vi "Multicast SubVI.vi"() -> (2 "nDevices":i32 caption="Найдено устройств", 3 "str":string[](array[string]))   [LabVIEW 2017, in "LV_Unicorn.lvlib"]
uses:
  LV_Unicorn.lvlib
  <vilib>/Utility/error.llb/DialogType.ctl
  Control/AnswerUDP.ctl
  GlobalMulticast.vi
  <vilib>/Utility/tcp.llb/UDP Multicast Read-Write Open.vi
panel:
  out "Array":string[][](array[string])
  out "modbustype, version":u32=4294967295 format="%08x"
  out "net address":u32
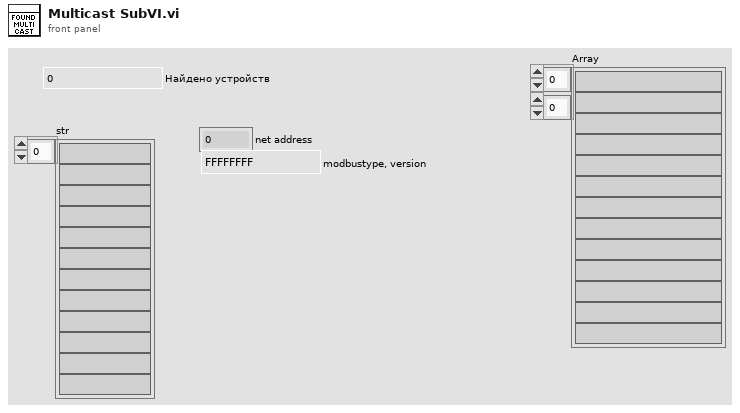
[diagram p1: front panel]
types:
  T1 = typedef "LV_Unicorn.lvlib/AnswerUDP.ctl" = cluster{"IP":string, "Port":u16, "DataVersion":u16, "ModbusAddress":i32, "type_version":string, "Description":string, "Serial":string, "ServerPort":u16}
  T2 = typedef "DialogType.ctl" = u16
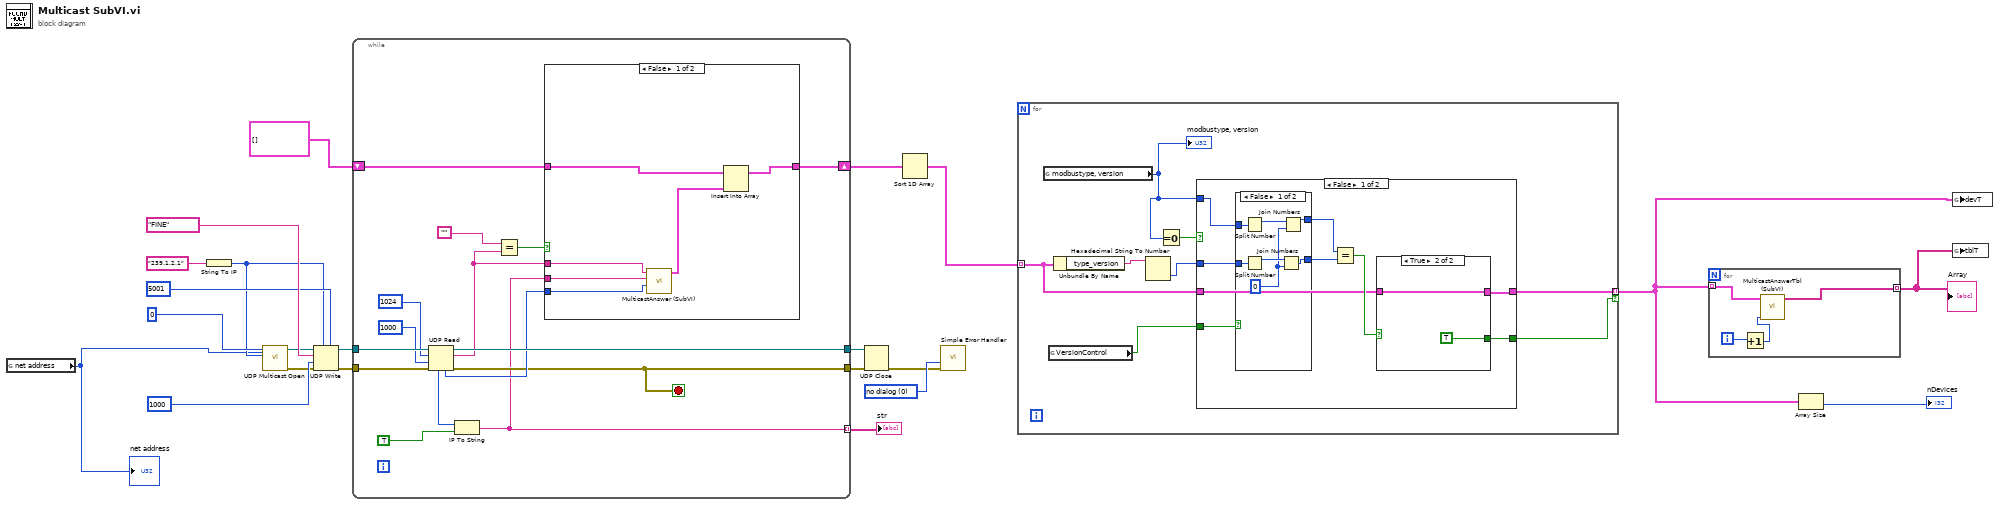
[diagram p0: block diagram]
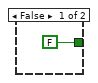
[diagram p3: hidden frame]
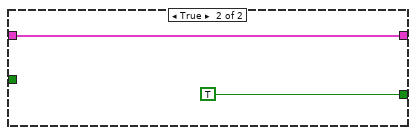
[diagram p4: hidden frame]
diagram:
  w17 = T2 0 items=["no dialog", "OK message", "continue or stop message", "OK message + warnings", "continue/stop + warnings"] ("type of dialog (OK msg:1)")
  n1 = global read "GlobalMulticast.vi" "net address"() -> (w1:u32)
  "net address" <- w1
  n2 = String To IP(1:"239.1.2.1" ("address")) -> (0:w12:u32)
  n3 = call-poly <vilib>:"UDP Multicast Open.vi"("net address"=w1, "multicast addr"=w12, "port"=u16 0) -> ("error out"=w13:errorcluster, "connection ID"=w14:refnum<k16>)  [unwired: 6 in, 1 out]
  n4 = UDP Write(address=w12, port or service name=u16 5001 ("port"), connection ID=w14, data in="FINE", 8:w13, 9:1000 ("timeout ms (25000)")) -> (error out=w9:errorcluster, 3:w11:refnum<k16>)
  n5 = while {
    tunnel: w11 -> [w37]
    tunnel: [w36] -> w10
    tunnel: w9 -> [w35]
    tunnel: [w28] -> w8
    tunnel: [w25] -> w22 mode=indexing
    shift-right: [w24] -> w7
    shift-left: T1[] [] -> [w23]
    stop <- w28 stop-if-true
    n6 = UDP Read(connection ID=w37, max size (548)=1024, timeout ms (25000)=1000, 8:w35) -> (data out=w31:string, error out=w28:errorcluster, 3:w36:refnum<k16>, 4:w30:u16, 6:w27:u32)
    n7 = IP To String(1:TRUE ("dot notation? (F)"), 2:w27) -> (0:w25:string)
    n8 = Equal?(x="", y=w31) -> (x = y?=w33:bool)
    n9 = case shown="False" w33 {
      tunnel: w31 -> [w43 _]
      tunnel: w25 -> [w42 _]
      tunnel: w30 -> [w41 _]
      tunnel: [w40 w44] -> w24
      tunnel: w23 -> [w39 w44]
      frame False {
        n10 = call "MulticastAnswer (SubVI).vi"("port"=w41, "name"=w42, "data in"=w43) -> ("SUdpAnswer"=w38:T1)  [unwired: 7 in, 1 out]
        n11 = Insert Into Array(array=w39, new element=w38) -> (w40:T1[])  [unwired: 1 in]
      }
      frame True {
      }
    }
  }
  "str" <- w22
  n12 = UDP Close(connection ID=w10, 8:w8) -> (error out=w15:errorcluster)  [unwired: 1 out]
  n13 = Sort 1D Array(array=w7) -> (sorted array=w6:T1[])
  n14 = call <vilib>:"Simple Error Handler.vi"("type of dialog (OK msg:1)"=w17, "error in (no error)"=w15) -> ()  [unwired: 3 in, 5 out]
  n15 = for {
    tunnel: w6 -> [w51] mode=indexing
    tunnel: [w50] -> w2 mode=indexing if=w49
    n16 = global read "GlobalMulticast.vi" "modbustype, version"() -> (w45:u32)
    "modbustype, version" <- w45
    n17 = global read "GlobalMulticast.vi" "VersionControl"() -> (w46:bool)
    n18 = Unbundle By Name(w51) -> ("type_version"=w48:string)
    n19 = Hexadecimal String To Number(string=w48) -> (number=w47:u32)  [unwired: 2 in, 1 out]
    n20 = Equal To 0?(x=w45) -> (x = 0?=w52:bool)
    n21 = case shown="False" w52 {
      tunnel: w51 -> [w60 w75]
      tunnel: [w59 w75] -> w50
      tunnel: w47 -> [w55 _]
      tunnel: [w58 TRUE] -> w49
      tunnel: w45 -> [w57 _]
      tunnel: w46 -> [w53 _]
      frame False {
        n22 = case shown="False" w53 {
          tunnel: w57 -> [w68 w70]
          tunnel: [w64 w70] -> w56
          tunnel: w55 -> [w67 w69]
          tunnel: [w62 w69] -> w54
          frame False {
            w63 = u16 0 ("lo")
            n23 = Split Number(x=w68) -> (hi(x)=w65:u16)  [unwired: 1 out]
            n24 = Split Number(x=w67) -> (hi(x)=w66:u16)  [unwired: 1 out]
            n25 = Join Numbers(hi=w66, lo=w63) -> ((hi.lo)=w62:u32)
            n26 = Join Numbers(hi=w65, lo=w63) -> ((hi.lo)=w64:u32)
          }
          frame True {
          }
        }
        n27 = Equal?(x=w56, y=w54) -> (x = y?=w61:bool)
        n28 = case shown="True" w61 {
          tunnel: w60 -> [_ w73]
          tunnel: [_ w73] -> w59
          tunnel: [FALSE TRUE] -> w58
          frame False {
          }
          frame True {
          }
        }
      }
      frame True {
      }
    }
  }
  n29 = for {
    tunnel: [w79] -> w3 mode=indexing
    tunnel: w2 -> [w78] mode=indexing
    i -> [w77]
    n30 = Increment(x=w77) -> (x+1=w76:i32)
    n31 = call "MulticastAnswerTbl (SubVI).vi"("count"=w76, "SUdpAnswer"=w78) -> ("Array"=w79:string[])  [unwired: 9 in]
  }
  "Array" <- w3
  n32 = Array Size(array=w2) -> (size(s)=→"nDevices":i32)
  n33 = global write "GlobalMulticast.vi" "devT"(w2) -> ()
  n34 = global write "GlobalMulticast.vi" "tblT"(w3) -> ()
